vi "Word_Insert_Chart.vi"(0 "AddOLEObject":refnum<k7>, 1 "measurement system":u16(ring) caption="measurement system (US)", 2 "Chart title":string, 5 "Data":dbl[][](array[numeric]) format="%.2f", 7 "Column header":string[](array[string]), 9 "Row header":string[](array[string]), 11 "error in":errorcluster, 12 "chart type":i32(ring)=51 items=["xlColumnClustered"=51, "xlColumnStacked"=52, "xlColumnStacked100"=53, "xl3DColumnClustered"=54, "xl3DColumnStacked"=55, "xl3DColumnStacked100"=56, "xlBarClustered"=57, "xlBarStacked"=58, "xlBarStacked100"=59, "xl3DBarClustered"=60, "xl3DBarStacked"=61, "xl3DBarStacked100"=62, "xlLineStacked"=63, "xlLineStacked100"=64, "xlLineMarkers"=65, "xlLineMarkersStacked"=66, "xlLineMarkersStacked100"=67, "xlPieOfPie"=68, "xlPieExploded"=69, "xl3DPieExploded"=70, "xlBarOfPie"=71, "xlXYScatterSmooth"=72, "xlXYScatterSmoothNoMarkers"=73, "xlXYScatterLines"=74, "xlXYScatterLinesNoMarkers"=75, "xlAreaStacked"=76, "xlAreaStacked100"=77, "xl3DAreaStacked"=78, "xl3DAreaStacked100"=79, "xlDoughnutExploded"=80, "xlRadarMarkers"=81, "xlRadarFilled"=82, "xlSurface"=83, "xlSurfaceWireframe"=84, "xlSurfaceTopView"=85, "xlSurfaceTopViewWireframe"=86, "xlBubble"=15, "xlBubble3DEffect"=87, "xlStockHLC"=88, "xlStockOHLC"=89, "xlStockVHLC"=90, "xlStockVOHLC"=91, "xlCylinderColClustered"=92, "xlCylinderColStacked"=93, "xlCylinderColStacked100"=94, "xlCylinderBarClustered"=95, "xlCylinderBarStacked"=96, "xlCylinderBarStacked100"=97, "xlCylinderCol"=98, "xlConeColClustered"=99, "xlConeColStacked"=100, "xlConeColStacked100"=101, "xlConeBarClustered"=102, "xlConeBarStacked"=103, "xlConeBarStacked100"=104, "xlConeCol"=105, "xlPyramidColClustered"=106, "xlPyramidColStacked"=107, "xlPyramidColStacked100"=108, "xlPyramidBarClustered"=109, "xlPyramidBarStacked"=110, "xlPyramidBarStacked100"=111, "xlPyramidCol"=112, "xl3DColumn"=-4100, "xlLine"=4, "xl3DLine"=-4101, "xl3DPie"=-4102, "xlPie"=5, "xlXYScatter"=-4169, "xl3DArea"=-4098, "xlArea"=1, "xlDoughnut"=-4120, "xlRadar"=-4151], 13 "chart size":cluster{"Height":i32, "Width":i32}={"Height"=300, "Width"=400}, 14 "has legend?":bool) -> (8 "start":i32, 10 "end":i32, 15 "error out":errorcluster)   [LabVIEW 2017, in "NI_ReportGenerationToolkit.lvlib"]
doc: "This VI opens Excel by creating an Automation Refnum for the Excel.Application object. Next it sets the \"Visible\" property to True/False depending on the Visible input."
uses:
  <vilib>/addons/_office/NI_ReportGenerationToolkit.lvlib
  <vilib>/Utility/NIReport.llb/NI_ReportGenerationCore.lvlib
panel:
  in  "Graph.Chart":refnum<k7>
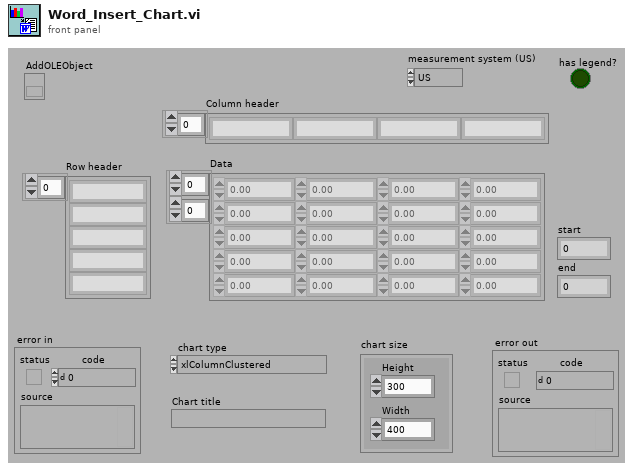
[diagram p1: front panel]
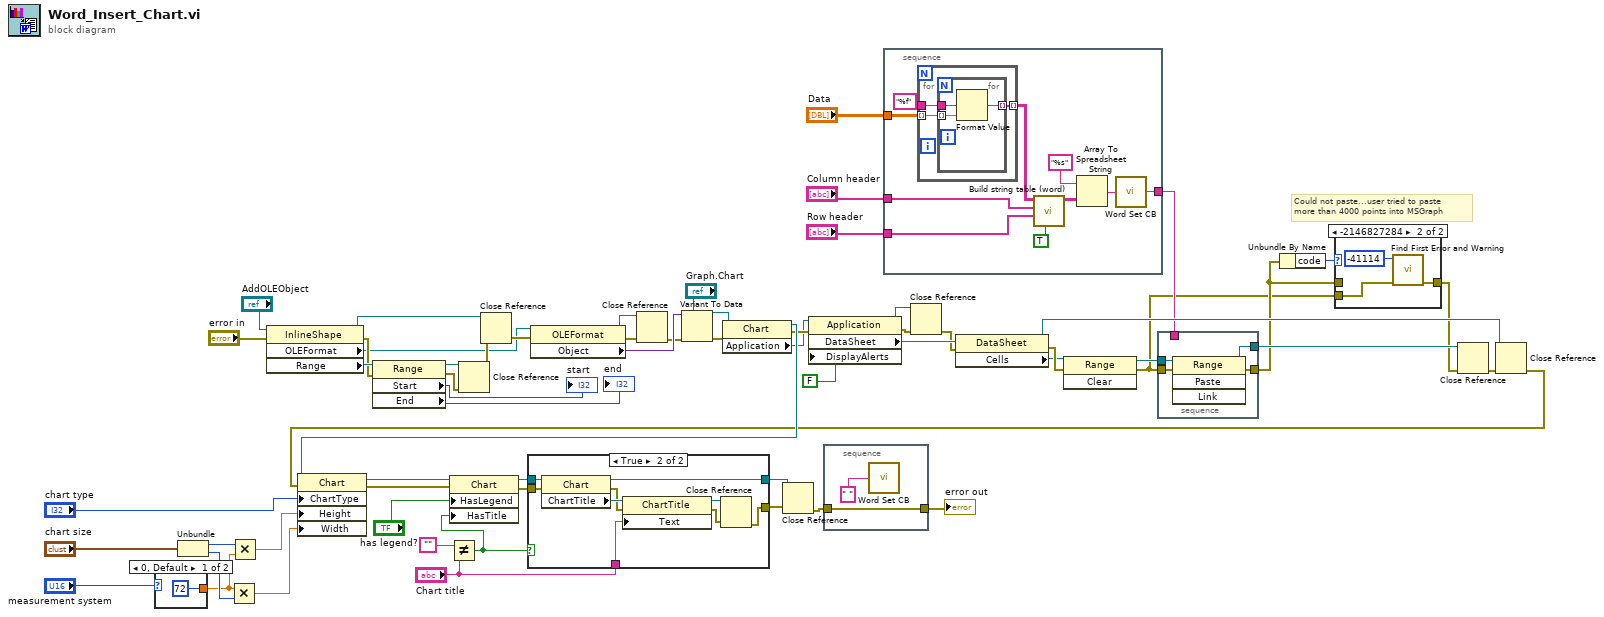
[diagram p0: block diagram]
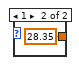
[diagram p3: hidden frame]
diagram:
  # "Could not paste...user tried to paste\nmore than 4000 points into MSGraph"
  n1 = case shown="0, Default" "measurement system" {
    tunnel: [72 28.35] -> w27
    frame 0, Default {
    }
    frame 1 {
    }
  }
  n2 = Unbundle("chart size") -> ("Height"=w28:i32, "Width"=w50:i32)
  n3 = Multiply(x=w27, y=w50) -> (x*y=w48:dbl)
  n4 = Multiply(x=w28, y=w27) -> (x*y=w49:dbl)
  n5 = property class="InlineShape"(reference="AddOLEObject", error in="error in") -> (reference out=w61:refnum<k7>, error out=w32:errorcluster, "OLEFormat"=w15:refnum<k7>, "Range"=w35:refnum<k7>)
  n6 = property class="Range"(reference=w35, error in=w32) -> (reference out=w33:refnum<k7>, error out=w34:errorcluster, "Start"=→"start":i32, "End"=→"end":i32)
  n7 = Not Equal?(x="", y="Chart title") -> (x != y?=w46:bool)
  n8 = Close Reference(reference=w33, error in (no error)=w34) -> (error out=w31:errorcluster)
  n9 = Close Reference(reference=w61, error in (no error)=w31) -> (error out=w16:errorcluster)
  n10 = property class="OLEFormat"(reference=w15, error in=w16) -> (reference out=w11:refnum<k7>, error out=w12:errorcluster, "Object"=w44:variant)
  n11 = Close Reference(reference=w11, error in (no error)=w12) -> (error out=w10:errorcluster)
  n12 = Variant To Data(error in=w10, type="Graph.Chart", Variant=w44) -> (data=w18:refnum<k7>, error out=w17:errorcluster)
  n13 = property class="Chart"(reference=w18, error in=w17) -> (reference out=w53:refnum<k7>, error out=w47:errorcluster, "Application"=w43:refnum<k7>)
  n14 = property class="Application"(reference=w43, error in=w47, "DisplayAlerts"=FALSE) -> (reference out=w7:refnum<k7>, error out=w8:errorcluster, "DataSheet"=w24:refnum<k7>)
  n15 = stacked-sequence {
    tunnel: "Data" -> [w74]
    tunnel: "Row header" -> [w73]
    tunnel: "Column header" -> [w66]
    tunnel: [w67] -> w21
    frame #0 {
      n16 = for {
        tunnel: w74 -> [w77] mode=indexing
        tunnel: "%f" -> [w76]
        tunnel: [w75] -> w72 mode=indexing
        n17 = for {
          tunnel: w77 -> [w80] mode=indexing
          tunnel: w76 -> [w79]
          tunnel: [w78] -> w75 mode=indexing
          n18 = Format Value(format string=w79, value (0)=w80) -> (output string=w78:string)  [unwired: 1 out]
        }
      }
      n19 = call <vilib>:"Build string table (word).vi"("Graph data?"=TRUE, "row headers"=w73, "column headers"=w66, "text data"=w72) -> ("output table"=w70:string[][])  [unwired: 7 out]
      n20 = Array To Spreadsheet String(array=w70, 3:"%s" ("format string")) -> (spreadsheet string=w68:string)  [unwired: 1 out]
      n21 = call <vilib>:"Word Set CB.vi"("String"=w68) -> ("String 2"=w67:string)
    }
  }
  n22 = Close Reference(reference=w7, error in (no error)=w8) -> (error out=w6:errorcluster)
  n23 = property class="DataSheet"(reference=w24, error in=w6) -> (reference out=w22:refnum<k7>, error out=w36:errorcluster, "Cells"=w20:refnum<k7>)
  n24 = invoke class="Range" method="Clear"(reference=w20, error in=w36) -> (reference out=w23:refnum<k7>, error out=w1:errorcluster)  [unwired: 1 in, 1 out]
  n25 = stacked-sequence {
    tunnel: [w84] -> w3
    tunnel: [w83] -> w41
    tunnel: w23 -> [w82]
    tunnel: w1 -> [w81]
    tunnel: w21 -> [_]
    frame #0 {
      n26 = invoke class="Range" method="Paste"(reference=w82, error in=w81) -> (reference out=w83:refnum<k7>, error out=w84:errorcluster)  [unwired: 2 in, 2 out]
    }
  }
  n27 = Unbundle By Name(w3) -> ("code"=w4:i32)
  n28 = case shown="-2146827284" w4 {
    tunnel: w3 -> [w85 _]
    tunnel: [w85 w88] -> w2
    tunnel: w1 -> [_ w86]
    frame Default {
    }
    frame -2146827284 {
      n29 = call <vilib>:"Find First Error and Warning.vi"("error in (no error)"=w86, "error code"=-41114) -> ("error out"=w88:errorcluster)  [unwired: 5 out]
    }
  }
  n30 = Close Reference(reference=w41, error in (no error)=w2) -> (error out=w40:errorcluster)
  n31 = Close Reference(reference=w22, error in (no error)=w40) -> (error out=w5:errorcluster)
  n32 = property class="Chart"(reference=w53, error in=w5, "ChartType"="chart type", "Height"=w49, "Width"=w48) -> (reference out=w59:refnum<k7>, error out=w58:errorcluster)
  n33 = property class="Chart"(reference=w59, error in=w58, "HasLegend"="has legend?", "HasTitle"=w46) -> (reference out=w57:refnum<k7>, error out=w56:errorcluster)
  n34 = case shown="True" w46 {
    tunnel: w57 -> [w89 w99]
    tunnel: w56 -> [w90 w97]
    tunnel: [w90 w93] -> w14
    tunnel: "Chart title" -> [_ w92]
    tunnel: [w89 w91] -> w13
    frame False {
    }
    frame True {
      n35 = property class="Chart"(reference=w99, error in=w97) -> (reference out=w91:refnum<k7>, error out=w96:errorcluster, "ChartTitle"=w98:refnum<k7>)
      n36 = property class="ChartTitle"(reference=w98, error in=w96, "Text"=w92) -> (reference out=w95:refnum<k7>, error out=w94:errorcluster)
      n37 = Close Reference(reference=w95, error in (no error)=w94) -> (error out=w93:errorcluster)
    }
  }
  n38 = Close Reference(reference=w13, error in (no error)=w14) -> (error out=w37:errorcluster)
  n39 = stacked-sequence {
    tunnel: w37 -> [w101]
    tunnel: [w101] -> w9
    frame #0 {
      n40 = call <vilib>:"Word Set CB.vi"("String"=" ") -> ()  [unwired: 1 out]
    }
  }
  "error out" <- w9
